vi "POST Multipart inputs to string log.vi"(11 "POST inputs":T1[](array[typedef])) -> (3 "POST inputs":string)   [LabVIEW 2020, in "Blue Easy HTTP OpenSource.lvlib"]
uses:
  Blue Easy HTTP OpenSource.lvlib
  <vilib>/httpClient/MultipartData.ctl
  <vilib>/Utility/error.llb/whitespace.ctl
  <vilib>/httpClient/LabVIEWHTTPClient.lvlib
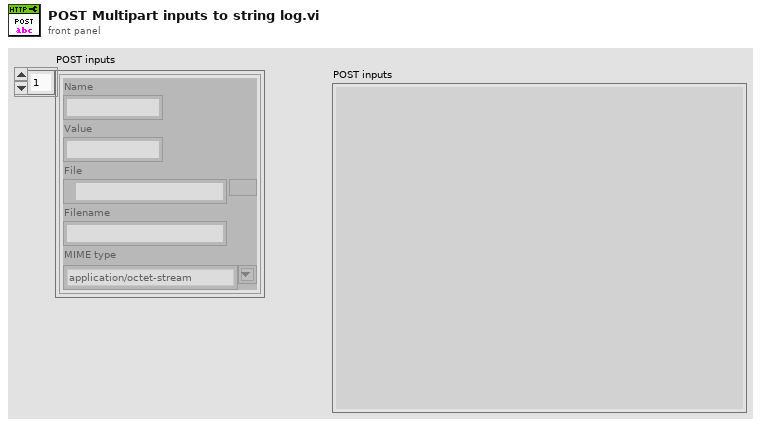
[diagram p1: front panel]
types:
  T1 = typedef "LabVIEWHTTPClient.lvlib/MultipartData.ctl" = cluster{"Name":string, "Value":string, "File":path, "Filename":string, "MIME type":string}
  T2 = typedef "whitespace.ctl" = u16
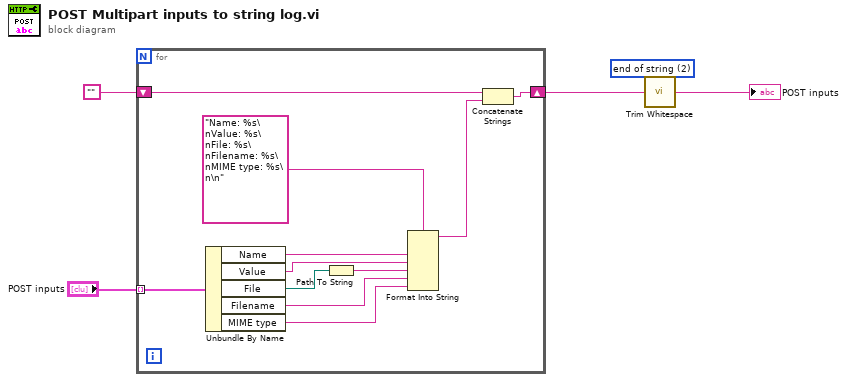
[diagram p0: block diagram]
diagram:
  w2 = T2 2 items=["both", "start of string", "end of string"] ("location (both)")
  n1 = for {
    tunnel: "POST inputs" -> [w16] mode=indexing
    shift-right: [w6] -> w3
    shift-left: "" -> [w8]
    n2 = Unbundle By Name(w16) -> ("Name"=w14:string, "Value"=w13:string, "File"=w12:path, "Filename"=w10:string, "MIME type"=w9:string)
    n3 = Path To String(path=w12) -> (string=w11:string)
    n4 = Format Into String(format string="Name: %s\nValue: %s\nFile: %s\nFilename: %s\nMIME type: %s\n\n", w14, w13, w11, w10, w9) -> (resulting string=w7:string)  [unwired: 2 in, 1 out]
    n5 = Concatenate Strings(w8, w7) -> (w6:string)
  }
  n6 = call <vilib>:"Trim Whitespace.vi"("string"=w3, "location (both)"=w2) -> ("trimmed string"=→"POST inputs":string)
